vi "RegisterSweep.vi"(8 "error in":errorcluster, 10 "RegisterSweepRoutedMessage":T2, 11 "config":T1) -> (0 "error out":errorcluster, 3 "config out":T1)   [LabVIEW 2017, in "EmsaDataEventCreator.lvlib"]
uses:
  <vilib>/addons/InsightCM/Devices/Shared/Emsa/EmsaDataEventCreator/EmsaDataEventCreator.lvlib
  <vilib>/addons/InsightCM/Devices/Shared/Emsa/EmsaDataEventCreator/controls/RegisterSweepRoutedMessage.ctl
  <vilib>/addons/InsightCM/Devices/Shared/Emsa/EmsaDataEventCreator/controls/Registry_Sweep.ctl
  <vilib>/addons/InsightCM/Devices/Shared/Common/DataEvent/controls/DataSetType.ctl
  <vilib>/addons/InsightCM/MessageBus/Base/controls/KeyValuePair.ctl
  <vilib>/addons/InsightCM/Devices/Shared/Emsa/EmsaDataEventCreator/controls/config.ctl
  <vilib>/addons/InsightCM/Devices/Shared/Emsa/EmsaDataEventCreator/controls/Registry.ctl
  <vilib>/addons/InsightCM/Devices/Shared/Common/DataEventCreator/controls/Registry_Trend.ctl
  <vilib>/addons/InsightCM/Devices/Shared/Common/DataEventCreator/DataEventCreator.lvlib
  <vilib>/addons/InsightCM/Devices/Shared/Common/DataEvent/DataEvent.lvlib
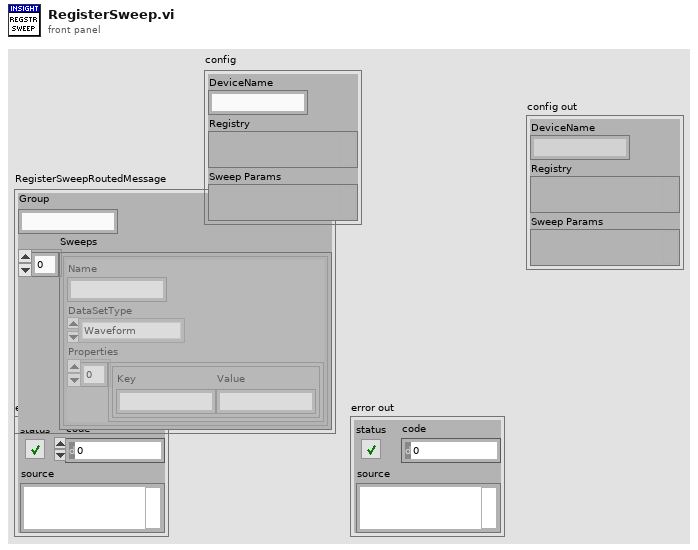
[diagram p1: front panel]
types:
  T1 = typedef "EmsaDataEventCreator.lvlib/config.ctl" = cluster{"DeviceName":string, "Registry":variant, "Sweep Params":variant}
  T2 = typedef "EmsaDataEventCreator.lvlib/RegisterSweepRoutedMessage.ctl" = cluster{"Group":string, "Sweeps":T3[]}
  T3 = typedef "EmsaDataEventCreator.lvlib/Registry_Sweep.ctl" = cluster{"Name":string, "DataSetType":T4, "Properties":T5[]}
  T4 = typedef "DataEvent.lvlib/DataSetType.ctl" = enum16{"Waveform", "SpeedProfile", "ThermalImage", "EmsaSweep"}
  T5 = typedef "KeyValuePair.ctl" = cluster{"Key":string, "Value":string}
  T6 = typedef "EmsaDataEventCreator.lvlib/Registry.ctl" = cluster{"Sweep Registry":T3[], "Trend Points":T7[], "AssetNodeMap":variant}
  T7 = typedef "DataEventCreator.lvlib/Registry_Trend.ctl" = cluster{"TrendPointId":string, "DataSetName":string, "HighRate":bool, "Always Send":bool}
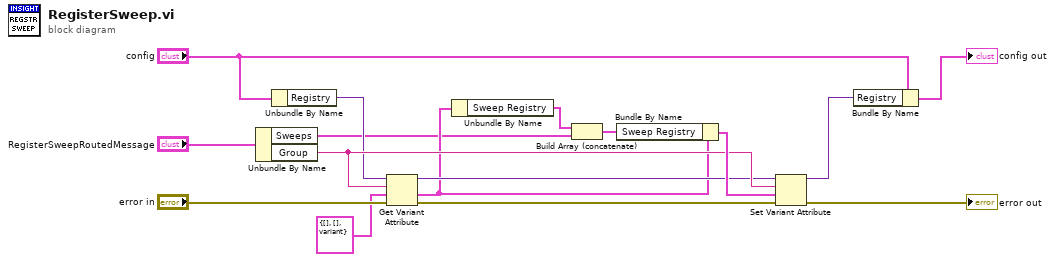
[diagram p0: block diagram]
diagram:
  n1 = Unbundle By Name("RegisterSweepRoutedMessage") -> ("Sweeps"=w2:T3[], "Group"=w14:string)
  n2 = Unbundle By Name("config") -> ("Registry"=w12:variant)
  n3 = Get Variant Attribute(Variant=w12, name=w14, default value (empty Variant)=T6 {"Sweep Registry"=[], "Trend Points"=[], "AssetNodeMap"=variant} ("Registry"), error in="error in") -> (duplicate Variant=w13:variant, value=w4:T6, error out=w16:errorcluster)  [unwired: 1 out]
  n4 = Unbundle By Name(w4) -> ("Sweep Registry"=w3:T3[])
  n5 = Build Array (concatenate)(w3, w2) -> (w1:T3[])
  n6 = Bundle By Name(cluster=w4, "Sweep Registry"=w1) -> (w15:T6)
  n7 = Set Variant Attribute(Variant=w13, name=w14, value=w15, error in=w16) -> (Variant out=w11:variant, error out=→"error out":errorcluster)  [unwired: 1 out]
  n8 = Bundle By Name(cluster="config", "Registry"=w11) -> (→"config out":T1)
